vi "Notify Match Successful.vi"(8 "error in":errorcluster, 11 "SDO Transfer in":refnum<class "SDO Transfer.lvclass">) -> (0 "error out":errorcluster, 3 "SDO Transfer out":refnum<class "SDO Transfer.lvclass">)   [LabVIEW 2020, in "CANopen.lvlib" / "SDO Manager.lvlib" / "SDO Transfer.lvclass"]
uses:
  SDO Transfer.lvclass
  SDO Transfer.lvclass/SDO Transfer.ctl
  SDO abort code.ctl
  Typedefs/SDO Result.ctl
  SDO Transfer Result.ctl
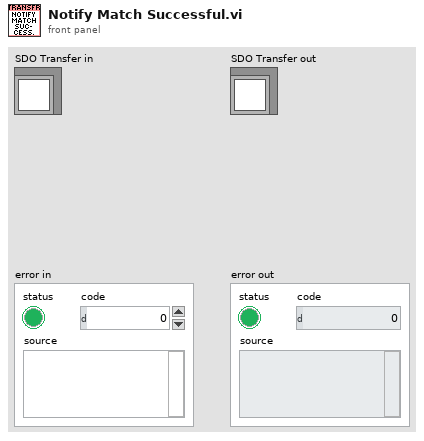
[diagram p1: front panel]
types:
  T1 = typedef "CANopen.lvlib/SDO Manager.lvlib/SDO Transfer.lvclass/SDO Transfer Result.ctl" = cluster{"SDO Result":T2, "Error":errorcluster}
  T2 = typedef "CANopen.lvlib/SDO Manager.lvlib/SDO Transfer.lvclass/SDO Result.ctl" = cluster{"Success":bool, "SDO abort code":cluster{"Null":bool, "Value":T3}, "Data":cluster{"Null":bool, "Data":u8[]}}
  T3 = typedef "CANopen.lvlib/SDO Manager.lvlib/SDO Transfer.lvclass/SDO abort code.ctl" = u32
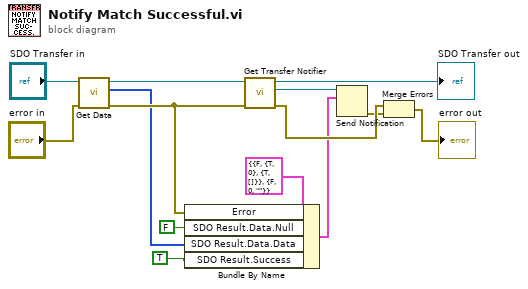
[diagram p0: block diagram]
diagram:
  n1 = call "Get Data.vi"("error in"="error in", "SDO Transfer in"="SDO Transfer in") -> ("error out"=w3:errorcluster, "Data"=w2:u8[], "SDO Transfer out"=w5:refnum<class "SDO Transfer.lvclass">)  [unwired: 7 in]
  n2 = Bundle By Name(cluster=T1 {"SDO Result"={"Success"=FALSE, "SDO abort code"={"Null"=TRUE, "Value"=0}, "Data"={"Null"=TRUE, "Data"=[]}}, "Error"={"status"=FALSE, "code"=0, "source"=""}} ("notification"), "Error"=w3, "SDO Result.Data.Null"=FALSE ("Data.Null"), "SDO Result.Data.Data"=w2, "SDO Result.Success"=TRUE) -> (w12:T1)
  n3 = call "Get Transfer Notifier.vi"("error in"=w3, "SDO Transfer in"=w5) -> ("error out"=w14:errorcluster, "SDO Transfer Notifier"=w8:refnum<notifier>, "SDO Transfer out"=→"SDO Transfer out":refnum<class "SDO Transfer.lvclass">)  [unwired: 7 in]
  n4 = Send Notification(notification=w12, notifier=w8) -> (error out=w6:errorcluster)  [unwired: 1 in, 1 out]
  n5 = Merge Errors(w14, w6) -> (→"error out":errorcluster)
